vi "Analysis.Result Summaries, Generate Pareto_V2.vi"(9 "Calc Duration":bool, 11 "ResultSum":T2[](array[typedef])) -> (0 "Test Time Histogram":T1(graph), 1 "Test Times (s)":cluster{"Min":dbl, "Max":dbl, "Avg":dbl}, 2 "Metrics":T3 {"Yield%" format="%.2f"}, 3 "FP Pareto":string[][](table))   [LabVIEW 2024]
uses:
  Analysis.Result Summary, Metrics.ctl
  Analysis.Result Summary_V2.ctl
  <vilib>/Analysis/NI_AALBase.lvlib
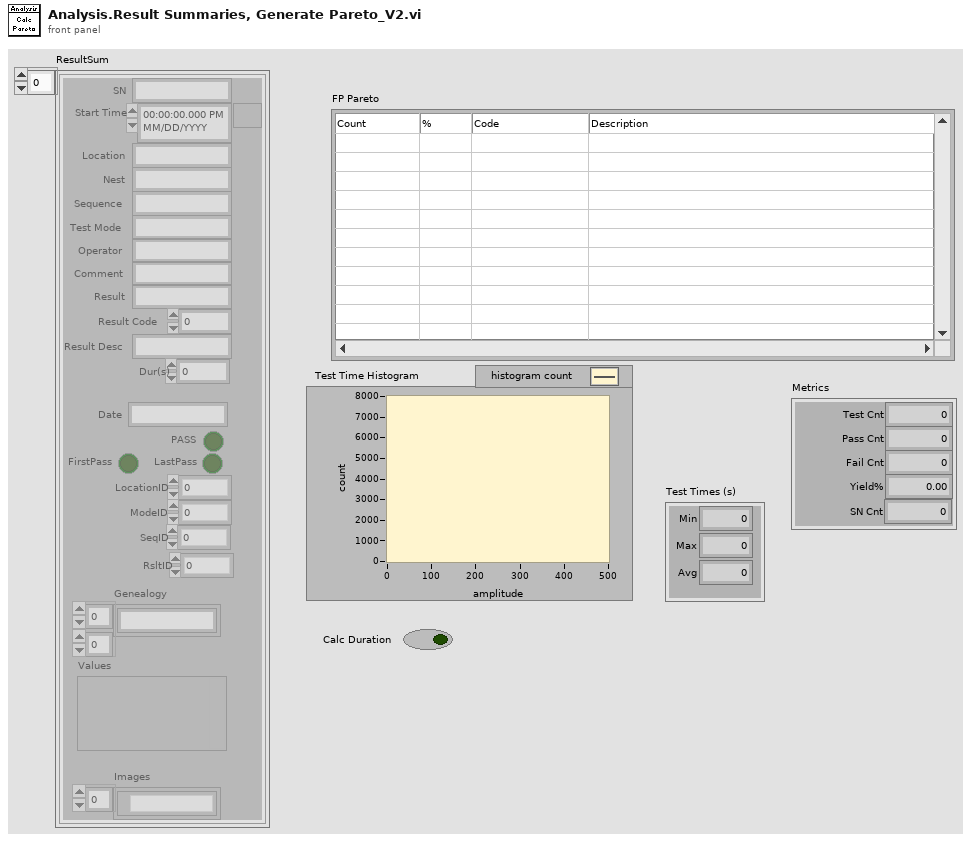
[diagram p1: front panel]
types:
  T1 = cluster{"X Values":dbl[], "Histogram: h(x)":i32[]}
  T2 = typedef "Analysis.Result Summary_V2.ctl" = cluster{"SN":string, "Start Time":timestamp, "Location":string, "Nest":string, "Sequence":string, "Operator":string, "Test Mode":string, "Comment":string, "Result":string, "Result Code":i32, "Result Desc":string, "Date":string, "Dur(s)":dbl, "PASS":bool, "FirstPass":bool, "LastPass":bool, "LocationID":i32, "ModeID":i32, "SeqID":i32, "RsltID":i32, "Genealogy":string[][], "Values":variant, "Images":path[]}
  T3 = typedef "Analysis.Result Summary, Metrics.ctl" = cluster{"Pass Cnt":i32, "Fail Cnt":i32, "Yield%":dbl, "Test Cnt":i32, "SN Cnt":i32}
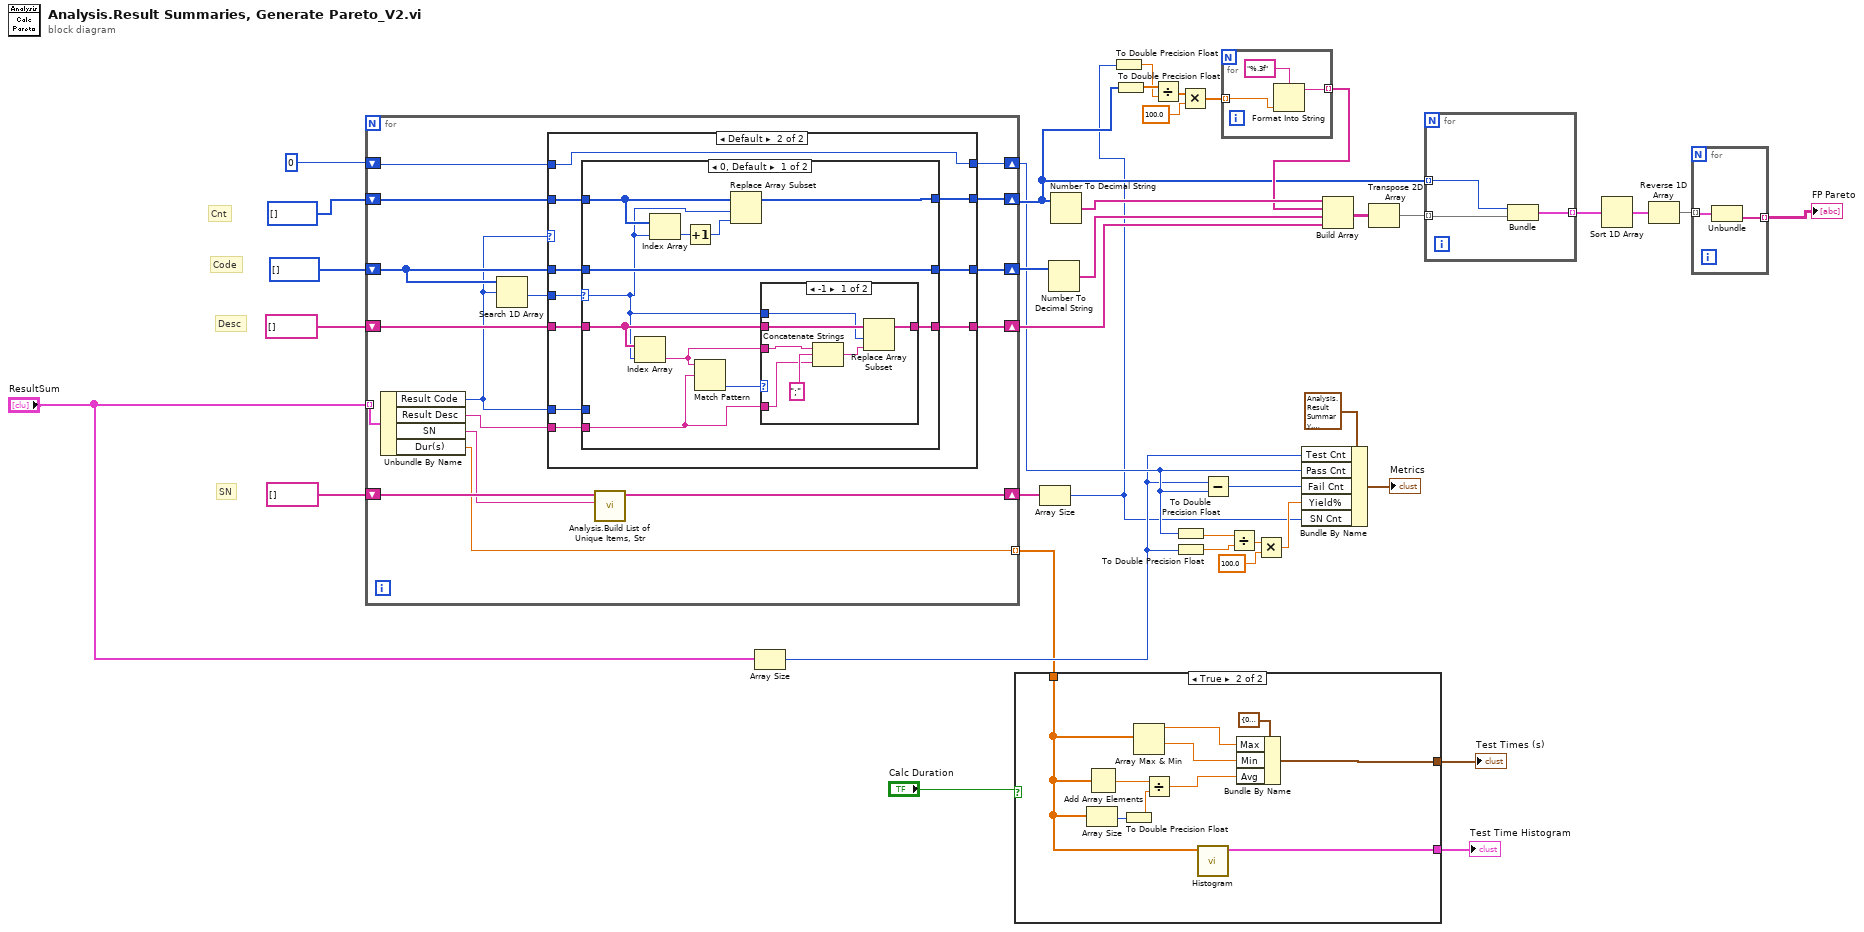
[diagram p0: block diagram]
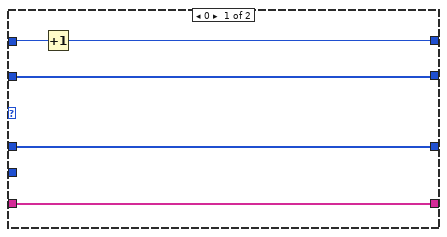
[diagram p3: hidden frame]
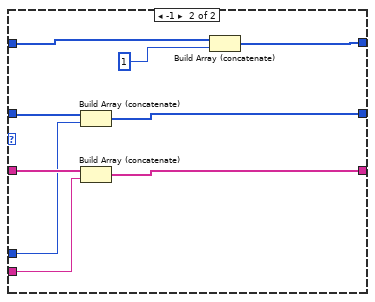
[diagram p5: hidden frame]
diagram:
  # "SN"
  # "Desc"
  # "Code"
  # "Cnt"
  n1 = for {
    shift-right: [w51] -> w23
    shift-left: i32[] [] -> [w54]
    shift-right: [w50] -> w20
    shift-left: i32[] [] -> [w53]
    shift-right: [w49] -> w36
    shift-left: string[] [] -> [w52]
    tunnel: "ResultSum" -> [w46] mode=indexing
    shift-right: [w47] -> w9
    shift-left: 0 ("Numeric") -> [w48]
    shift-right: [w41] -> w17
    shift-left: string[] [] -> [w43]
    tunnel: [w40] -> w5 mode=indexing
    n2 = Unbundle By Name(w46) -> ("Result Code"=w45:i32, "Result Desc"=w44:string, "SN"=w42:string, "Dur(s)"=w40:dbl)
    n3 = Search 1D Array(1D array=w53, element=w45) -> (index of element=w55:i32)  [unwired: 1 in]
    n4 = case shown="Default" w45 {
      tunnel: w55 -> [_ w70]
      tunnel: w54 -> [w60 w69]
      tunnel: w53 -> [w59 w68]
      tunnel: w52 -> [w58 w67]
      tunnel: [w60 w66] -> w51
      tunnel: [w59 w65] -> w50
      tunnel: [w58 w64] -> w49
      tunnel: w45 -> [_ w63]
      tunnel: w44 -> [_ w62]
      tunnel: w48 -> [w57 w61]
      tunnel: [w56 w61] -> w47
      frame 0 {
        n5 = Increment(x=w57) -> (x+1=w56:i32)
      }
      frame Default {
        n6 = case shown="0, Default" w70 {
          selector: w70 -> [w71 _]
          tunnel: w69 -> [w80 w95]
          tunnel: w68 -> [w77 w97]
          tunnel: w67 -> [w75 w98]
          tunnel: [w81 w94] -> w66
          tunnel: [w77 w93] -> w65
          tunnel: [w74 w92] -> w64
          tunnel: w63 -> [_ w90]
          tunnel: w62 -> [w72 w91]
          frame 0, Default {
            n7 = Index Array(array=w75, index=w71) -> (element=w73:string)
            n8 = Index Array(array=w80, index=w71) -> (element=w79:i32)
            n9 = Increment(x=w79) -> (x+1=w78:i32)
            n10 = Match Pattern(string=w73, regular expression=w72) -> (offset past match=w76:i32)  [unwired: 1 in, 3 out]
            n11 = Replace Array Subset(array=w80, new element=w78, index=w71) -> (w81:i32[])
            n12 = case shown="-1" w76 {
              tunnel: w75 -> [w87 w89]
              tunnel: [w88 w89] -> w74
              tunnel: w73 -> [w86 _]
              tunnel: w72 -> [w84 _]
              tunnel: w71 -> [w82 _]
              frame -1 {
                n13 = Concatenate Strings(w86, ";", w84) -> (w83:string)
                n14 = Replace Array Subset(array=w87, new element=w83, index=w82) -> (w88:string[])
              }
              frame Default {
              }
            }
          }
          frame -1 {
            n15 = Build Array (concatenate)(w97, w90) -> (w93:i32[])
            n16 = Build Array (concatenate)(w98, w91) -> (w92:string[])
            n17 = Build Array (concatenate)(w95, 1) -> (w94:i32[])
          }
        }
      }
    }
    n18 = call "Analysis.Build List of Unique Items, Str.vi"("Item In"=w42, "List In"=w43) -> ("List Out"=w41:string[])  [unwired: 7 in, 2 out]
  }
  n19 = Array Size(array="ResultSum") -> (size(s)=w6:i32)
  n20 = case shown="True" "Calc Duration" {
    tunnel: w5 -> [_ w105]
    tunnel: [_ w100] -> w2
    tunnel: [_ w99] -> w1
    frame False {
    }
    frame True {
      n21 = Array Size(array=w105) -> (size(s)=w106:i32)
      n22 = Add Array Elements(numeric array=w105) -> (sum=w108:dbl)
      n23 = To Double Precision Float(number=w106) -> (double precision float=w107:dbl)
      n24 = Array Max & Min(array=w105) -> (max value=w101:dbl, min value=w102:dbl)  [unwired: 2 out]
      n25 = Divide(x=w108, y=w107) -> (x/y=w103:dbl)
      n26 = call <vilib>:"Histogram.vi"("X"=w105) -> ("Histogram Graph"=w99:T1)  [unwired: 7 in, 3 out]
      n27 = Bundle By Name(cluster=cluster{"Min":dbl, "Max":dbl, "Avg":dbl} {"Min"=0.0, "Max"=0.0, "Avg"=0.0} ("Test Times (s)"), "Max"=w101, "Min"=w102, "Avg"=w103) -> (w100:cluster{"Min":dbl, "Max":dbl, "Avg":dbl})
    }
  }
  "Test Times (s)" <- w2
  "Test Time Histogram" <- w1
  n28 = Array Size(array=w17) -> (size(s)=w4:i32)
  n29 = Number To Decimal String(number=w20) -> (decimal integer string=w19:string[])  [unwired: 1 in]
  n30 = Number To Decimal String(number=w23) -> (decimal integer string=w25:string[])  [unwired: 1 in]
  n31 = To Double Precision Float(number=w4) -> (double precision float=w21:dbl)
  n32 = To Double Precision Float(number=w23) -> (double precision float=w22:dbl[])
  n33 = Divide(x=w22, y=w21) -> (x/y=w26:dbl[])
  n34 = To Double Precision Float(number=w9) -> (double precision float=w12:dbl)
  n35 = To Double Precision Float(number=w6) -> (double precision float=w13:dbl)
  n36 = Multiply(x=w26, y=100.0) -> (x*y=w28:dbl[])
  n37 = Subtract(x=w6, y=w9) -> (x-y=w14:i32)
  n38 = for {
    tunnel: w28 -> [w110] mode=indexing
    tunnel: [w109] -> w24 mode=indexing
    n39 = Format Into String(format string="%.3f", w110) -> (resulting string=w109:string)  [unwired: 2 in, 1 out]
  }
  n40 = Divide(x=w12, y=w13) -> (x/y=w11:dbl)
  n41 = Multiply(x=w11, y=100.0) -> (x*y=w8:dbl)
  n42 = Bundle By Name(cluster=T3 {"Pass Cnt"=5050, "Fail Cnt"=374, "Yield%"=93.1047197640118, "Test Cnt"=5424, "SN Cnt"=374} ("Metrics"), "Test Cnt"=w6, "Pass Cnt"=w9, "Fail Cnt"=w14, "Yield%"=w8, "SN Cnt"=w4) -> (→"Metrics":T3)
  n43 = Build Array(w25, w24, w19, w36) -> (w35:string[][])
  n44 = Transpose 2D Array(2D array=w35) -> (transposed array=w34:string[][])
  n45 = for {
    tunnel: w34 -> [w112] mode=indexing
    tunnel: w23 -> [w114] mode=indexing
    tunnel: [w113] -> w32 mode=indexing
    n46 = Bundle("Numeric"=w114, w112) -> (w113:cluster{"Numeric":i32, string[]})  [unwired: 1 in]
  }
  n47 = Sort 1D Array(array=w32) -> (sorted array=w31:cluster{"Numeric":i32, string[]}[])
  n48 = Reverse 1D Array(array=w31) -> (reversed array=w30:cluster{"Numeric":i32, string[]}[])
  n49 = for {
    tunnel: w30 -> [w116] mode=indexing
    tunnel: [w115] -> w29 mode=indexing
    n50 = Unbundle(w116) -> (w115:string[])  [unwired: 1 out]
  }
  "FP Pareto" <- w29
